vi "Handle getAll.vi"(8 "error in (no error)":errorcluster, 11 "Inst.Krohn-Hite-7008 in":refnum<class "Inst.Krohn-Hite-7008.lvclass">) -> (0 "error out":errorcluster, 2 "getAll":variant, 3 "Inst.Krohn-Hite-7008 out":refnum<class "Inst.Krohn-Hite-7008.lvclass">)   [LabVIEW 2019, in "Inst.Krohn-Hite-7008.lvclass"]
uses:
  Inst.Krohn-Hite-7008.lvclass
  Inst.Krohn-Hite-7008.lvclass/Inst.Krohn-Hite-7008.ctl
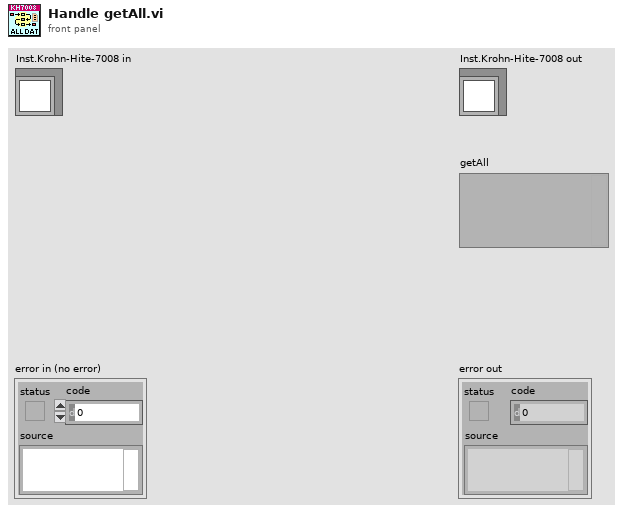
[diagram p1: front panel]
types:
  T1 = typedef "Inst.Krohn-Hite-7008.lvclass/Inst.Krohn-Hite-7008.getAll--Cluster.ctl" = cluster{"device_id":string, "model":string, "channelParameters(json)":string, "allChannelProperties":T2}
  T2 = typedef "KH7008.lvlib/allChannelProperties--Array.ctl" = T3[]
  T3 = typedef "KH7008.lvlib/channelProperties--Cluster.ctl" = cluster{"Channel":T4, "Gain":T5, "Input":T6, "Shunt":T7, "Coupling":T8, "Filter":T9}
  T4 = typedef "KH7008.lvlib/Channel--Enum.ctl" = enum8{"Channel 1", "Channel 2", "Channel 3", "Channel 4", "Channel 5", "Channel 6", "Channel 7", "Channel 8"}
  T5 = typedef "KH7008.lvlib/Gain--Enum.ctl" = enum8{"1x", "10x", "100x", "1000x"}
  T6 = typedef "KH7008.lvlib/Input--Enum.ctl" = enum8{"OFF", "SE+", "SE-", "DIFF"}
  T7 = typedef "KH7008.lvlib/Shunt--Enum.ctl" = enum8{"Open", "50 Ohms", "500 Ohms", "5k Ohms", "50k Ohms", "10M Ohm"}
  T8 = typedef "KH7008.lvlib/Coupling--Enum.ctl" = enum8{"AC", "DC"}
  T9 = typedef "KH7008.lvlib/Filter--Enum.ctl" = enum8{"OFF", "ON"}
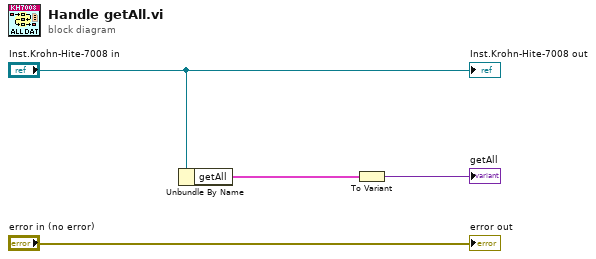
[diagram p0: block diagram]
diagram:
  n1 = Unbundle By Name("Inst.Krohn-Hite-7008 in") -> ("getAll"=w4:T1)
  n2 = To Variant(anything=w4) -> (Variant=→"getAll":variant)
  "error out" <- "error in (no error)"
  "Inst.Krohn-Hite-7008 out" <- "Inst.Krohn-Hite-7008 in"
